vi "TEST_SpecCheck.vi"(8 "Level in":dbl=3.635000000000013 format="%#_13g", 11 "Spec Range In":T1={"Specs"=[3.735, 3.635, 4.085, 1011.0, 989.0, 910.0, 890.0], "LUT Status"={"ChA/!ChB"=FALSE, "Drain/!Fill"=FALSE, "In Range?"=TRUE, "Switch Range?"=FALSE, "Measure R?"=FALSE, "Vaild R?"=TRUE, "Index(n)"=10, "Index(n-1)"=9, "Index Max"=13}}) -> (3 "Spec Range Out":T1={"Specs"=[3.735, 3.635, 4.085, 1011.0, 989.0, 910.0, 890.0], "LUT Status"={"ChA/!ChB"=FALSE, "Drain/!Fill"=FALSE, "In Range?"=TRUE, "Switch Range?"=TRUE, "Measure R?"=FALSE, "Vaild R?"=FALSE, "Index(n)"=10, "Index(n-1)"=9, "Index Max"=13}})   [LabVIEW 2024]
uses:
  Control Definitions/Def Spec RNG.ctl
  Control Definitions/Ded LUT_Status.ctl
panel:
  in  "stop":bool
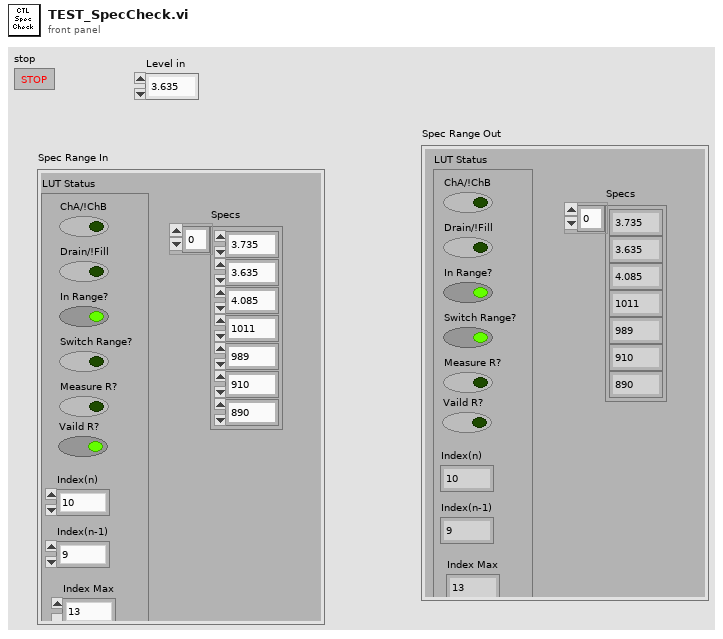
[diagram p1: front panel]
types:
  T1 = typedef "Def Spec RNG.ctl" = cluster{"Specs":dbl[], "LUT Status":T2}
  T2 = typedef "Ded LUT_Status.ctl" = cluster{"ChA/!ChB":bool, "Drain/!Fill":bool, "In Range?":bool, "Switch Range?":bool, "Measure R?":bool, "Vaild R?":bool, "Index(n)":i32, "Index(n-1)":i32, "Index Max":i32}
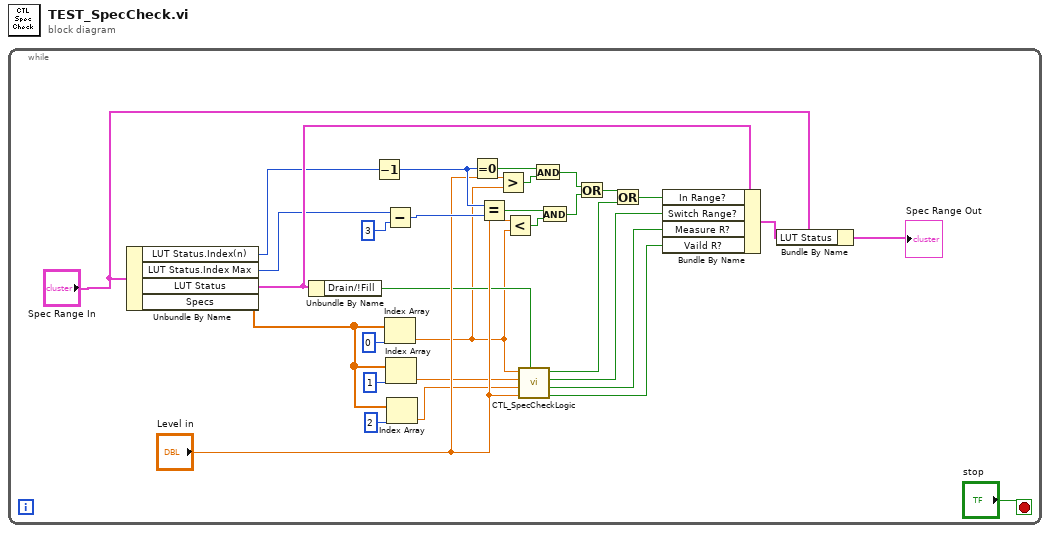
[diagram p0: block diagram]
diagram:
  n1 = while {
    stop <- "stop" stop-if-true
    n2 = Unbundle By Name("Spec Range In") -> ("LUT Status.Index(n)"=w9:i32, "LUT Status.Index Max"=w10:i32, "LUT Status"=w13:T2, "Specs"=w31:dbl[])
    n3 = Unbundle By Name(w13) -> ("Drain/!Fill"=w6:bool)
    n4 = Decrement(x=w9) -> (x-1=w29:i32)
    n5 = Subtract(x=w10, y=3) -> (x-y=w24:i32)
    n6 = Index Array(array=w31, index=0) -> (element=w5:dbl)
    n7 = Index Array(array=w31, index=1) -> (element=w4:dbl)
    n8 = Index Array(array=w31, index=2) -> (element=w3:dbl)
    n9 = Equal To 0?(x=w29) -> (x = 0?=w20:bool)
    n10 = Equal?(x=w29, y=w24) -> (x = y?=w18:bool)
    n11 = Greater?(x="Level in", y=w5) -> (0:w19:bool)
    n12 = Less?(x="Level in", y=w5) -> (x < y?=w17:bool)
    n13 = call "CTL_SpecCheckLogic.vi"("Drain!Fill In"=w6, "Level in"="Level in", "Spec Hi(n+1)"=w3, "Spec Lo (n)"=w4, "Spec Hi (n)"=w5) -> ("Vaild R?"=w8:bool, "Measure R?"=w2:bool, "Switch Range?"=w28:bool, "In Range?"=w26:bool)  [unwired: 2 in, 1 out]
    n14 = And(x=w20, y=w19) -> (x .and. y?=w22:bool)
    n15 = And(x=w18, y=w17) -> (x .and. y?=w21:bool)
    n16 = Or(x=w22, y=w21) -> (x .or. y?=w25:bool)
    n17 = Or(x=w25, y=w26) -> (x .or. y?=w27:bool)
    n18 = Bundle By Name(cluster=w13, "In Range?"=w27, "Switch Range?"=w28, "Measure R?"=w2, "Vaild R?"=w8) -> (w30:T2)
    n19 = Bundle By Name(cluster="Spec Range In", "LUT Status"=w30) -> (→"Spec Range Out":T1)
  }
